vi "Do Task.vi"(8 "error in":errorcluster, 9 "Input":variant, 10 "Task Ident":string, 11 "Series Actor in":refnum<class "Series Actor.lvclass">) -> (0 "error out":errorcluster, 3 "Series Actor out":refnum<class "Series Actor.lvclass">)   [LabVIEW 2023, in "Series Actor.lvlib" / "Series Actor.lvclass"]
uses:
  Series Actor.lvclass
  Series Actor.lvclass/Series Actor.ctl
  Task/ITask Actor/ITask Actor Messages/Do Msg/Do Msg.lvclass/Do Msg.ctl
  <vilib>/ActorFramework/Message Enqueuer/Message Enqueuer.lvclass/Message Enqueuer.ctl
  <vilib>/ActorFramework/Message Enqueuer/Enqueue.vi
  Task/ITask Actor/ITask Actor Messages/Do Msg/Do Msg.lvclass
  <vilib>/Utility/error.llb/Error Cluster From Error Code.vi
  <vilib>/Utility/LVClass/Get LV Class Name.vi
  <resource>/AFDebug/Generate Trace for Message.vi
  <vilib>/ActorFramework/Message Priority Queue/Priority Enqueue.vi
  <vilib>/ErrorRing/Error Ring.xnode
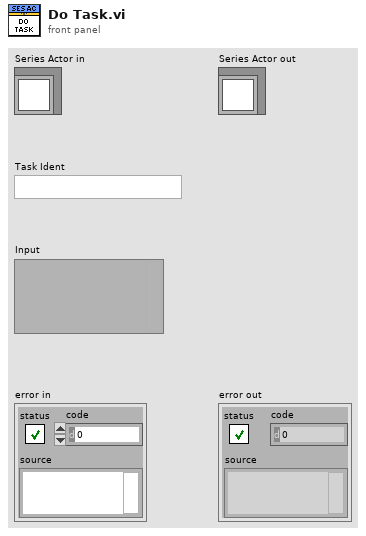
[diagram p1: front panel]
types:
  T1 = map{string, refnum<class "Message Enqueuer.lvclass">}
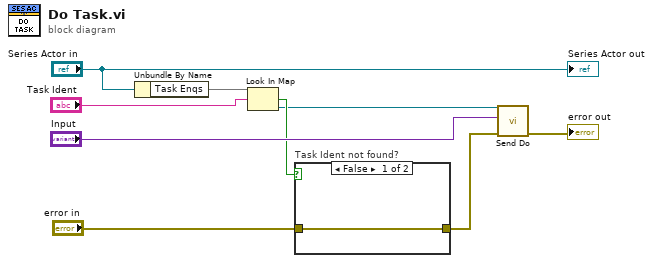
[diagram p0: block diagram]
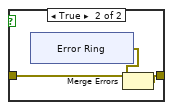
[diagram p2: hidden frame]
diagram:
  n1 = Unbundle By Name("Series Actor in") -> ("Task Enqs"=w4:T1)
  n2 = Look In Map(map=w4, key="Task Ident") -> (key not found?=w3:bool, value=w1:refnum<class "Message Enqueuer.lvclass">)  [unwired: 1 in]
  n3 = case "Task Ident not found?" shown="False" w3 {
    tunnel: "error in" -> [w10 w13]
    tunnel: [w10 w11] -> w2
    frame False {
    }
    frame True {
      n4 = xnode "Error Ring"() -> ("error out"=w12:errorcluster)
      n5 = Merge Errors(w13, w12) -> (w11:errorcluster)
    }
  }
  n6 = call "Send Do.vi"("error in (no error)"=w2, "Input"="Input", "Message Enqueuer"=w1) -> ("error out"=→"error out":errorcluster)  [unwired: 7 in, 1 out]
  "Series Actor out" <- "Series Actor in"
